vi "雷达流速仪通讯.vi"(6 "Slave ID":u8=1, 7 "STEP":enum16{"open", "read", "write", "close"}(ring)=enum."read", 8 "Error in":errorcluster caption="Error in (no error)", 9 "values":u16[](array[numeric]), 10 "quantity":u16, 11 "starting address":u16 format="%.0x") -> (0 "error out":errorcluster, 2 "输出簇":T1, 3 "Registers":u16[](array[numeric]))   [LabVIEW 2016, in "雷达流速仪.lvlib"]
uses:
  <vilib>/Plasmionique/MB Master/MB_ADU/MB_ADU.lvclass/MB_ADU.ctl
  <vilib>/Plasmionique/MB Master/MB_ADU/Read RX Data.vi
  <vilib>/Plasmionique/MB Master/MB_ADU/Read RX Timestamp.vi
  <vilib>/Plasmionique/MB Master/MB_ADU/Read Slave ID.vi
  <vilib>/Plasmionique/MB Master/MB_ADU/Read TX Data.vi
  <vilib>/Plasmionique/MB Master/MB_ADU/Read TX Timestamp.vi
  <vilib>/Plasmionique/MB Master/MB_Master_Serial/MB_Master_Serial.lvclass
  C:/Program Files (x86)/National Instruments/LabVIEW 2016/vi.lib/Plasmionique/MB Master/MB_Master/MB_Master.lvclass
  <vilib>/Plasmionique/MB Master/MB_ADU/MB_ADU.lvclass
  <vilib>/Plasmionique/MB Master/MB Master.lvlib
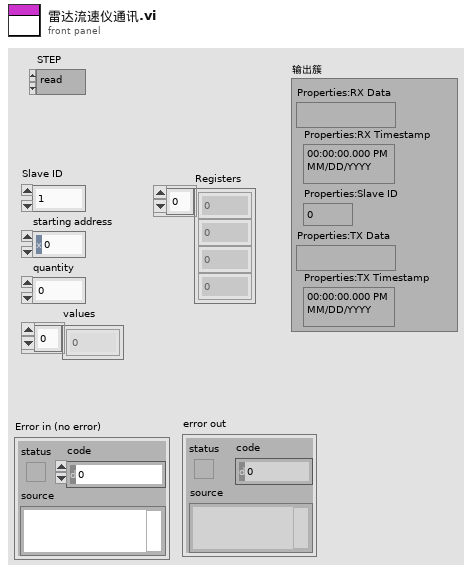
[diagram p1: front panel]
types:
  T1 = cluster{"Properties:RX Data":string, "Properties:RX Timestamp":timestamp, "Properties:Slave ID":u8, "Properties:TX Data":string, "Properties:TX Timestamp":timestamp}
  T2 = cluster{"baud rate (bps)":u32, "stop bits":u16, "parity":u16, "flow control":u16, "timeout":u32, "retries":i32}
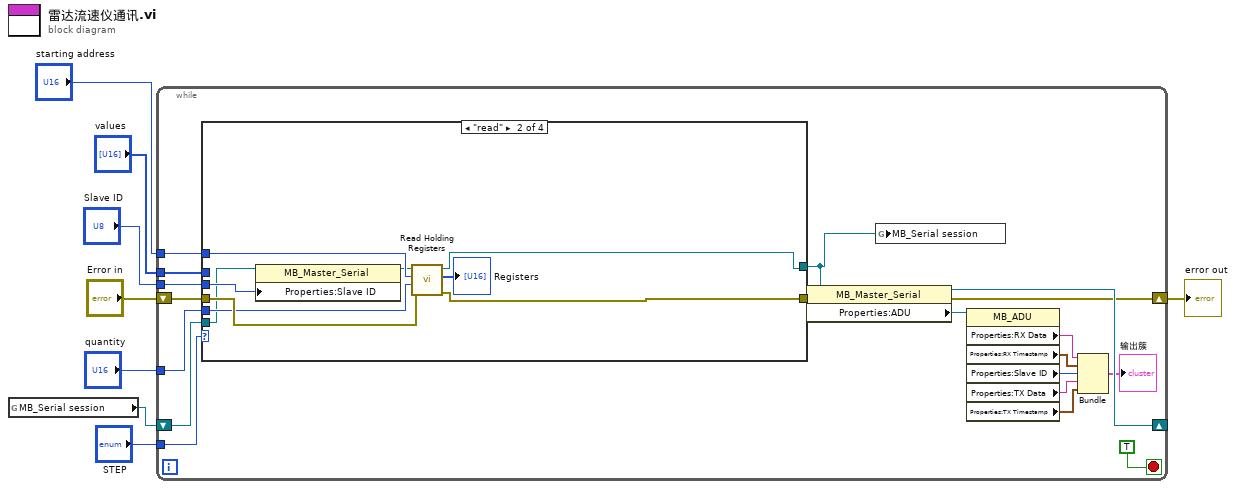
[diagram p0: block diagram]
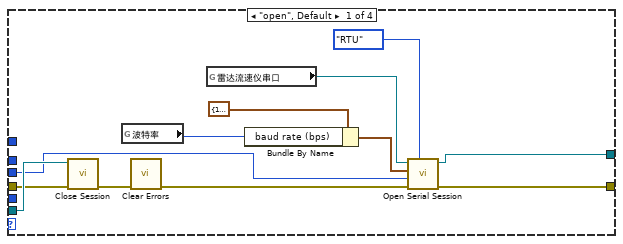
[diagram p2: hidden frame]
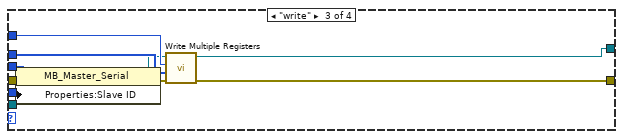
[diagram p3: hidden frame]
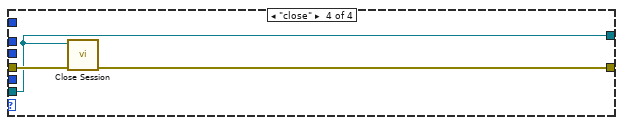
[diagram p4: hidden frame]
diagram:
  n1 = global read "雷达流速仪全局变量.vi" "MB_Serial session"() -> (w1:refnum<class "MB_Master_Serial.lvclass">)
  n2 = while {
    shift-right: [w21] -> _
    shift-left: w1 -> [w27]
    shift-right: [w19] -> w7
    shift-left: "Error in" -> [w26]
    tunnel: "Slave ID" -> [w25]
    tunnel: "starting address" -> [w24]
    tunnel: "quantity" -> [w23]
    tunnel: "STEP" -> [w22]
    tunnel: "values" -> [w12]
    stop <- TRUE stop-if-true
    n3 = case shown="\"read\"" w22 {
      tunnel: w27 -> [w37 w41 w53 w58]
      tunnel: w26 -> [w36 w48 w50 w60]
      tunnel: [w28 w47 w56 w58] -> w9
      tunnel: [w38 w46 w57 w59] -> w20
      tunnel: w25 -> [w33 w44 w52 _]
      tunnel: w24 -> [_ w43 w55 _]
      tunnel: w23 -> [_ w42 _ _]
      tunnel: w12 -> [_ _ w54 _]
      frame "open", Default {
        n4 = call-dynamic "Close Session.vi"("error in (no error)"=w36, "MB_Serial session"=w37) -> ("error out"=w32:errorcluster)  [unwired: 9 in]
        n5 = global read "雷达流速仪全局变量.vi" "波特率"() -> (w29:u32)
        n6 = call <vilib>:"Clear Errors.vi"("error in (no error)"=w32) -> ("error out"=w31:errorcluster)  [unwired: 5 in, 1 out]
        n7 = global read "雷达流速仪全局变量.vi" "雷达流速仪串口"() -> (w30:refnum<visa-resource-name>)
        n8 = Bundle By Name(cluster=T2 {"baud rate (bps)"=115200, "stop bits"=10, "parity"=0, "flow control"=0, "timeout"=500, "retries"=1} ("Serial Config"), "baud rate (bps)"=w29) -> (w34:T2)
        n9 = call <vilib>:"Open Serial Session.vi"("Mode (RTU)"=enum16{"RTU", "ASCII"}."RTU", "Error in"=w31, "Slave ID"=w33, "Serial Config"=w34, "VISA Resource"=w30) -> ("Error out"=w38:errorcluster, "MB_Serial session"=w28:refnum<class "MB_Master_Serial.lvclass">)  [unwired: 5 in]
      }
      frame "read" {
        n10 = property class="MB_Master_Serial"(reference=w41, "Properties:Slave ID"=w44) -> (reference out=w40:refnum<class "MB_Master_Serial.lvclass">)  [unwired: 1 in, 1 out]
        n11 = call <vilib>:"Read Holding Registers.vi"("error in (no error)"=w48, "quantity"=w42, "starting address"=w43, "MB session in"=w40) -> ("error out"=w46:errorcluster, "Registers"=→"Registers":u16[], "MB session out"=w47:refnum<class "MB_Master_Serial.lvclass">)  [unwired: 5 in]
      }
      frame "write" {
        n12 = property class="MB_Master_Serial"(reference=w53, error in=w50, "Properties:Slave ID"=w52) -> (reference out=w51:refnum<class "MB_Master_Serial.lvclass">, error out=w49:errorcluster)
        n13 = call <vilib>:"Write Multiple Registers.vi"("error in (no error)"=w49, "values"=w54, "starting address"=w55, "MB session in"=w51) -> ("error out"=w57:errorcluster, "MB session out"=w56:refnum<class "MB_Master_Serial.lvclass">)  [unwired: 6 in]
      }
      frame "close" {
        n14 = call-dynamic "Close Session.vi"("error in (no error)"=w60, "MB_Serial session"=w58) -> ("error out"=w59:errorcluster)  [unwired: 9 in]
      }
    }
    n15 = property class="MB_Master_Serial"(reference=w9, error in=w20) -> (reference out=w21:refnum<class "MB_Master_Serial.lvclass">, error out=w19:errorcluster, "Properties:ADU"=w10:refnum<class "MB_ADU.lvclass">)
    n16 = global write "雷达流速仪全局变量.vi" "MB_Serial session"(w9) -> ()
    n17 = property class="MB_ADU"(reference=w10) -> ("Properties:RX Data"=w18:string, "Properties:RX Timestamp"=w17:timestamp, "Properties:Slave ID"=w16:u8, "Properties:TX Data"=w15:string, "Properties:TX Timestamp"=w14:timestamp)  [unwired: 1 in, 2 out]
    n18 = Bundle("Properties:RX Data"=w18, "Properties:RX Timestamp"=w17, "Properties:Slave ID"=w16, "Properties:TX Data"=w15, "Properties:TX Timestamp"=w14) -> (→"输出簇":T1)  [unwired: 1 in]
  }
  "error out" <- w7
